vi "setPhase.vi"(8 "error in (no error)":errorcluster, 10 "phase":dbl, 11 "rf in":refnum<class "rf.lvclass">) -> (0 "error out":errorcluster, 3 "rf out":refnum<class "rf.lvclass">)   [LabVIEW 2009, in "Tools.lvlib" / "Scripting.lvlib" / "rf.lvclass"]
uses:
  rf.lvclass
  rf.lvclass/rf.ctl
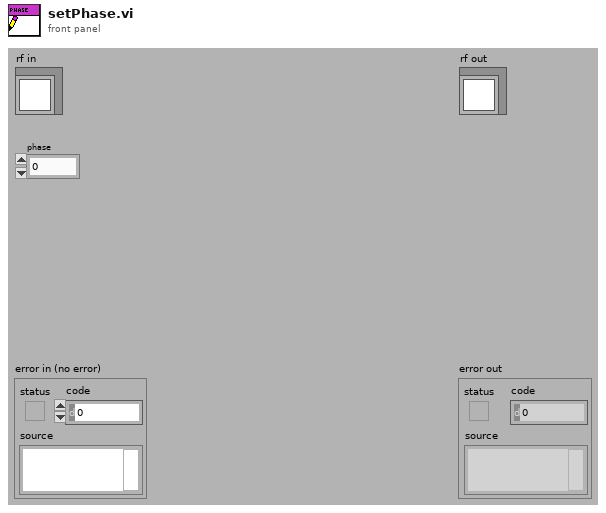
[diagram p1: front panel]
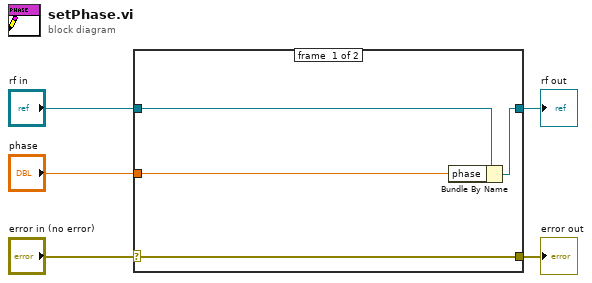
[diagram p0: block diagram]
diagram:
  n1 = case shown="No Error" "error in (no error)" {
    selector: "error in (no error)" -> [w9 w10]
    tunnel: [w9 w10] -> w4
    tunnel: [w7 w11] -> w2
    tunnel: "rf in" -> [w8 w11]
    tunnel: "phase" -> [w6 _]
    frame #0 {
      n2 = Bundle By Name(cluster=w8, "phase"=w6) -> (w7:refnum<class "rf.lvclass">)
    }
    frame #1 {
    }
  }
  "error out" <- w4
  "rf out" <- w2
